vi "SJA_Query.vi"(0 "System no.":i32=1 min=1 max=4 step=1, 3 "Invert order?":bool=TRUE, 5 "error in":errorcluster) -> (14 "Axis 1":string, 15 "Axis 2":string, 19 "error out":errorcluster)   [LabVIEW 2020]
doc: "Indicates which axes can be controlled with a joystick connected to the controller.\n\nC-848: Invert order? must be TRUE\nC-880: Invert order? must be TRUE"
uses:
  Syntax.ctl
  Global1.vi
panel:
  # "Indicates which axes can be controlled with a joystick \nconnected to the controller."
  # "Joystick controlled"
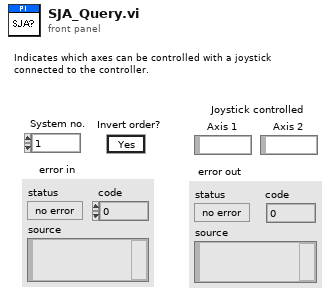
[diagram p1: front panel]
types:
  T1 = typedef "Syntax.ctl" = enum16{"GCS 1.0", "GCS 2.0", "GCS 3.0"}
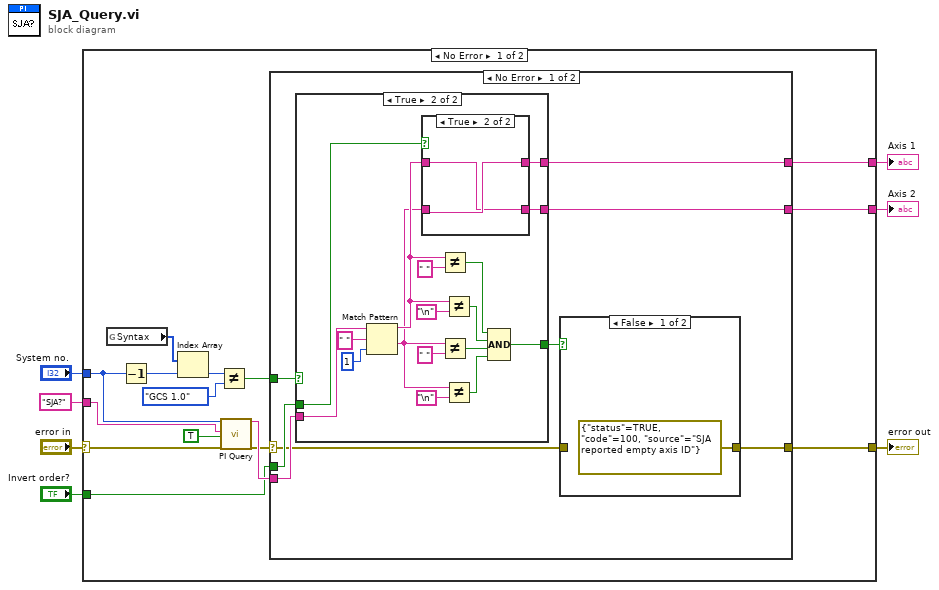
[diagram p0: block diagram]
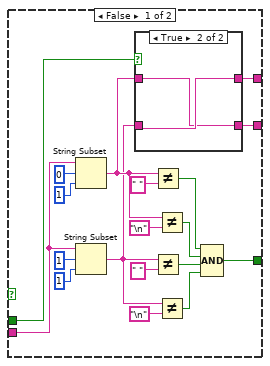
[diagram p2: hidden frame]
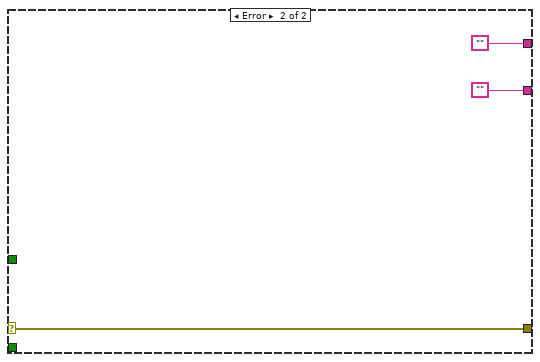
[diagram p6: hidden frame]
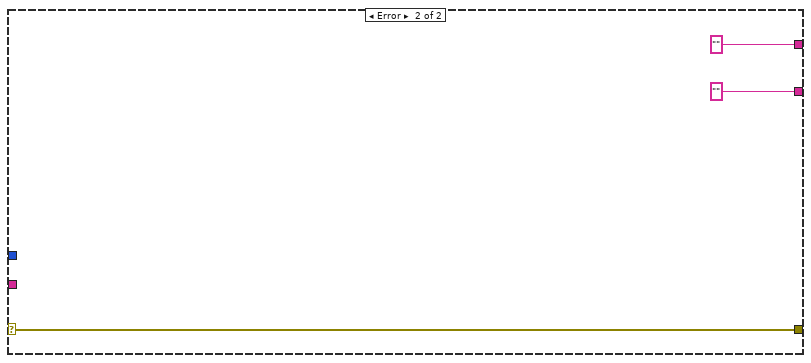
[diagram p7: hidden frame]
diagram:
  n1 = case shown="No Error" "error in" {
    selector: "error in" -> [w12 w80]
    tunnel: "SJA?" -> [w22 _]
    tunnel: "System no." -> [w14 _]
    tunnel: [w20 ""] -> w5
    tunnel: [w19 ""] -> w4
    tunnel: [w18 w80] -> w3
    tunnel: "Invert order?" -> [w10 _]
    frame No Error {
      n2 = global read "Global1.vi" "Syntax"() -> (w15:T1[])
      n3 = Decrement(x=w14) -> (x-1=w16:i32)
      n4 = Index Array(array=w15, index=w16) -> (element=w17:T1)
      n5 = Not Equal?(x=w17, y=Syntax."GCS 1.0") -> (x != y?=w13:bool)
      n6 = call "PI Query.vi"("System no."=w14, "String to send"=w22, "Attach termination char.?"=TRUE ("Attach Linefeed?"), "error in"=w12) -> ("String read"=w11:string, "error out"=w9:errorcluster)  [unwired: 3 in, 11 out]
      n7 = case shown="No Error" w9 {
        selector: w9 -> [w23 w77]
        tunnel: w11 -> [w30 _]
        tunnel: [w26 ""] -> w20
        tunnel: [w25 ""] -> w19
        tunnel: [w28 w77] -> w18
        tunnel: w10 -> [w27 _]
        tunnel: w13 -> [w24 _]
        frame No Error {
          n8 = case shown="True" w24 {
            tunnel: w30 -> [w41 w58]
            tunnel: [w36 w62] -> w29
            tunnel: w27 -> [w35 w61]
            tunnel: [w34 w60] -> w26
            tunnel: [w32 w59] -> w25
            frame False {
              n9 = String Subset(string=w41, offset (0)=0, length (rest)=1 ("length")) -> (substring=w33:string)
              n10 = String Subset(string=w41, offset (0)=1, length (rest)=1 ("length")) -> (substring=w31:string)
              n11 = case shown="True" w35 {
                tunnel: [w51 w53] -> w34
                tunnel: w33 -> [w51 w52]
                tunnel: [w50 w52] -> w32
                tunnel: w31 -> [w50 w53]
                frame False {
                }
                frame True {
                }
              }
              n12 = Not Equal?(x=w33, y=" ") -> (x != y?=w40:bool)
              n13 = Not Equal?(x=w31, y=" ") -> (x != y?=w38:bool)
              n14 = Not Equal?(x=w33, y="\n") -> (x != y?=w39:bool)
              n15 = Not Equal?(x=w31, y="\n") -> (x != y?=w37:bool)
              n16 = Compound Arithmetic op=AND(w40, w39, w38, w37) -> (w36:bool)
            }
            frame True {
              n17 = Match Pattern(string=w58, regular expression=" ", offset (0)=1) -> (before substring=w55:string, after substring=w54:string)  [unwired: 2 out]
              n18 = case shown="True" w61 {
                tunnel: [w72 w74] -> w60
                tunnel: w55 -> [w72 w73]
                tunnel: [w71 w73] -> w59
                tunnel: w54 -> [w71 w74]
                frame False {
                }
                frame True {
                }
              }
              n19 = Not Equal?(x=w55, y=" ") -> (x != y?=w66:bool)
              n20 = Not Equal?(x=w54, y=" ") -> (x != y?=w64:bool)
              n21 = Not Equal?(x=w55, y="\n") -> (x != y?=w65:bool)
              n22 = Not Equal?(x=w54, y="\n") -> (x != y?=w63:bool)
              n23 = Compound Arithmetic op=AND(w66, w65, w64, w63) -> (w62:bool)
            }
          }
          n24 = case shown="False" w29 {
            tunnel: [errorcluster {"status"=TRUE, "code"=100, "source"="SJA reported empty axis ID"} ("error out") w76] -> w28
            tunnel: w23 -> [_ w76]
            frame False {
            }
            frame True {
            }
          }
        }
        frame Error {
        }
      }
    }
    frame Error {
    }
  }
  "error out" <- w3
  "Axis 1" <- w5
  "Axis 2" <- w4
